vi "Get_Set_Buttons.vi"(8 "Status/Errors in":refnum<vi>, 9 "Set?":T1, 10 "Main parameters":T3={"Mode"={"Mode"=enum."Dialog", "Expert?"=FALSE, "Dialog?"=FALSE}, "Stop loop"={"Settings changed?"=FALSE, "Stop?"=refnum}, "Send message"={"Send mode"=enum."Get parameters", "Set parameter list"=0, "Get parameter list"=0, "Reset device"=0, "Length set settings message"=0, "Reset buttons?"=FALSE, "Reset Master?"=enum."General"}, "Write settings"={"Options"=enum."File 1"}, "Settings state"={"MAS locked?"=refnum, "SLV locked?"=refnum}, "Button refs"={"Stop program"=refnum, "Save settings"=refnum, "DAQ mode"=refnum, "Reset settings"=refnum, "Apply settings"=refnum, "Reset MAS"=refnum, "Reset SLV"=refnum, "Local DBase?"=refnum, "Last value DBase"=FALSE, "Database"=refnum, "Calibration"=refnum, "Save settings 2"=refnum}, "Update screen"={"Detector number"=0, "Hardware"=enum."None"}, "Files"={"Path config file"=path "", "Path def. ini file"=path "", "Path ini file 1"=path "", "Path ini file 2"=path "", "Path RBF file"=path ""}, "DB connection"={"connection reference"=refnum, "Connected?"=refnum, "ODBC Name"=""}, "Status_id"=refnum, "Time difference"=refnum, "Satellites"=refnum, "Alignment parameters"=refnum, "Page Statistics 2"=refnum, "Database"=refnum, "Page Statistics"=refnum} {"Update screen"."Detector number" format="%#.0f"; "Send message"."Reset device" format="%x"; "Send message"."Get parameter list" format="%x"; "Send message"."Set parameter list" format="%x"}) -> (0 "Status/Errors out":refnum<vi>, 1 "Button values":T2 caption="Buttons", 2 "Enabled State Expert":u8, 3 "Enabled State Normal":u8, 4 "Calibration value":bool, 5 "DAQ mode value":bool)   [LabVIEW 2013]
uses:
  Controls/Main_Parameters.ctl
  Controls/Mode.ctl
  Controls/Stop_Loop.ctl
  Controls/Send_Message.ctl
  Controls/Send_Message_Mode.ctl
  Controls/Master.ctl
  Controls/Write_Settings.ctl
  Controls/Write_Settings_Options.ctl
  Controls/Settings_State.ctl
  Controls/Button_Refs.ctl
  Controls/Update_Screen.ctl
  Controls/Files.ctl
  Controls/DB_Connection.ctl
  database/Connection.llb/Conn ObjectReference.ctl
  Controls/Button_Values.ctl
  Controls/Get_Set_Buttons_mode.ctl
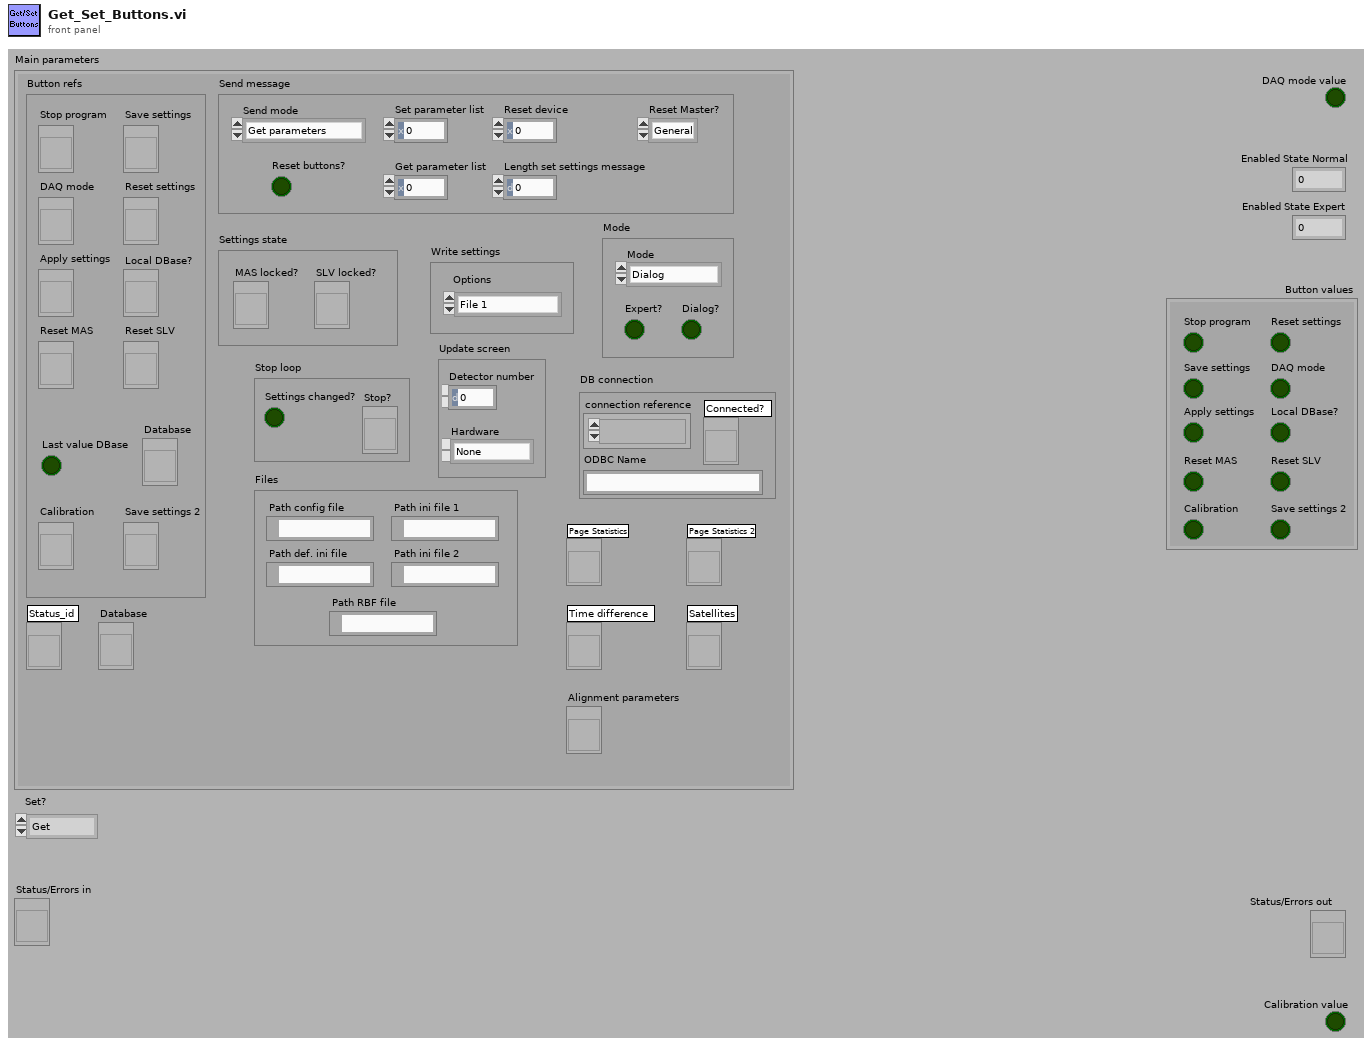
[diagram p1: front panel]
types:
  T1 = typedef "Get_Set_Buttons_mode.ctl" = enum16{"Get", "Get DAQ", "Set", "Set settings"}
  T2 = typedef "Button_Values.ctl" = cluster{"Stop program":bool, "Save settings":bool, "Apply settings":bool, "Reset settings":bool, "DAQ mode":bool, "Reset MAS":bool, "Reset SLV":bool, "Local DBase?":bool, "Calibration":bool, "Save settings 2":bool}
  T3 = typedef "Main_Parameters.ctl" = cluster{"Mode":T4, "Stop loop":T5, "Send message":T6, "Write settings":T9, "Settings state":T11, "Button refs":T12, "Update screen":T13, "Files":T14, "DB connection":T15, "Status_id":refnum<vi>, "Time difference":refnum<vi>, "Satellites":refnum<vi>, "Alignment parameters":refnum<vi>, "Page Statistics 2":refnum<vi>, "Database":refnum<vi>, "Page Statistics":refnum<vi>}
  T4 = typedef "Mode.ctl" = cluster{"Mode":enum8{"Stop", "Dialog", "Hisparc II", "Hisparc II DAQ", "Alignment"}, "Expert?":bool, "Dialog?":bool}
  T5 = typedef "Stop_Loop.ctl" = cluster{"Settings changed?":bool, "Stop?":refnum<vi>}
  T6 = typedef "Send_Message.ctl" = cluster{"Send mode":T7, "Set parameter list":u8, "Get parameter list":u8, "Reset device":u8, "Length set settings message":i32, "Reset buttons?":bool, "Reset Master?":T8}
  T7 = typedef "Send_Message_Mode.ctl" = enum16{"Get parameters", "Set parameters", "From front panel", "From parameters", "Reset device", "Alignment"}
  T8 = typedef "Master.ctl" = enum16{"Master", "Slave", "General"}
  T9 = typedef "Write_Settings.ctl" = cluster{"Options":T10}
  T10 = typedef "Write_Settings_Options.ctl" = enum16{"File 1", "File 2", "Alignment", "Reset"}
  T11 = typedef "Settings_State.ctl" = cluster{"MAS locked?":refnum<vi>, "SLV locked?":refnum<vi>}
  T12 = typedef "Button_Refs.ctl" = cluster{"Stop program":refnum<vi>, "Save settings":refnum<vi>, "DAQ mode":refnum<vi>, "Reset settings":refnum<vi>, "Apply settings":refnum<vi>, "Reset MAS":refnum<vi>, "Reset SLV":refnum<vi>, "Local DBase?":refnum<vi>, "Last value DBase":bool, "Database":refnum<vi>, "Calibration":refnum<vi>, "Save settings 2":refnum<vi>}
  T13 = typedef "Update_Screen.ctl" = cluster{"Detector number":u16, "Hardware":enum8{"None", "HiSPARC I", "HiSPARC II", "HiSPARC III", "Unknown"}}
  T14 = typedef "Files.ctl" = cluster{"Path config file":path, "Path def. ini file":path, "Path ini file 1":path, "Path ini file 2":path, "Path RBF file":path}
  T15 = typedef "DB_Connection.ctl" = cluster{"connection reference":T16, "Connected?":refnum<vi>, "ODBC Name":string}
  T16 = typedef "Conn ObjectReference.ctl" = refnum<k1>
  T17 = enum8{"Stop", "Dialog", "Hisparc II", "Hisparc II DAQ", "Alignment"}
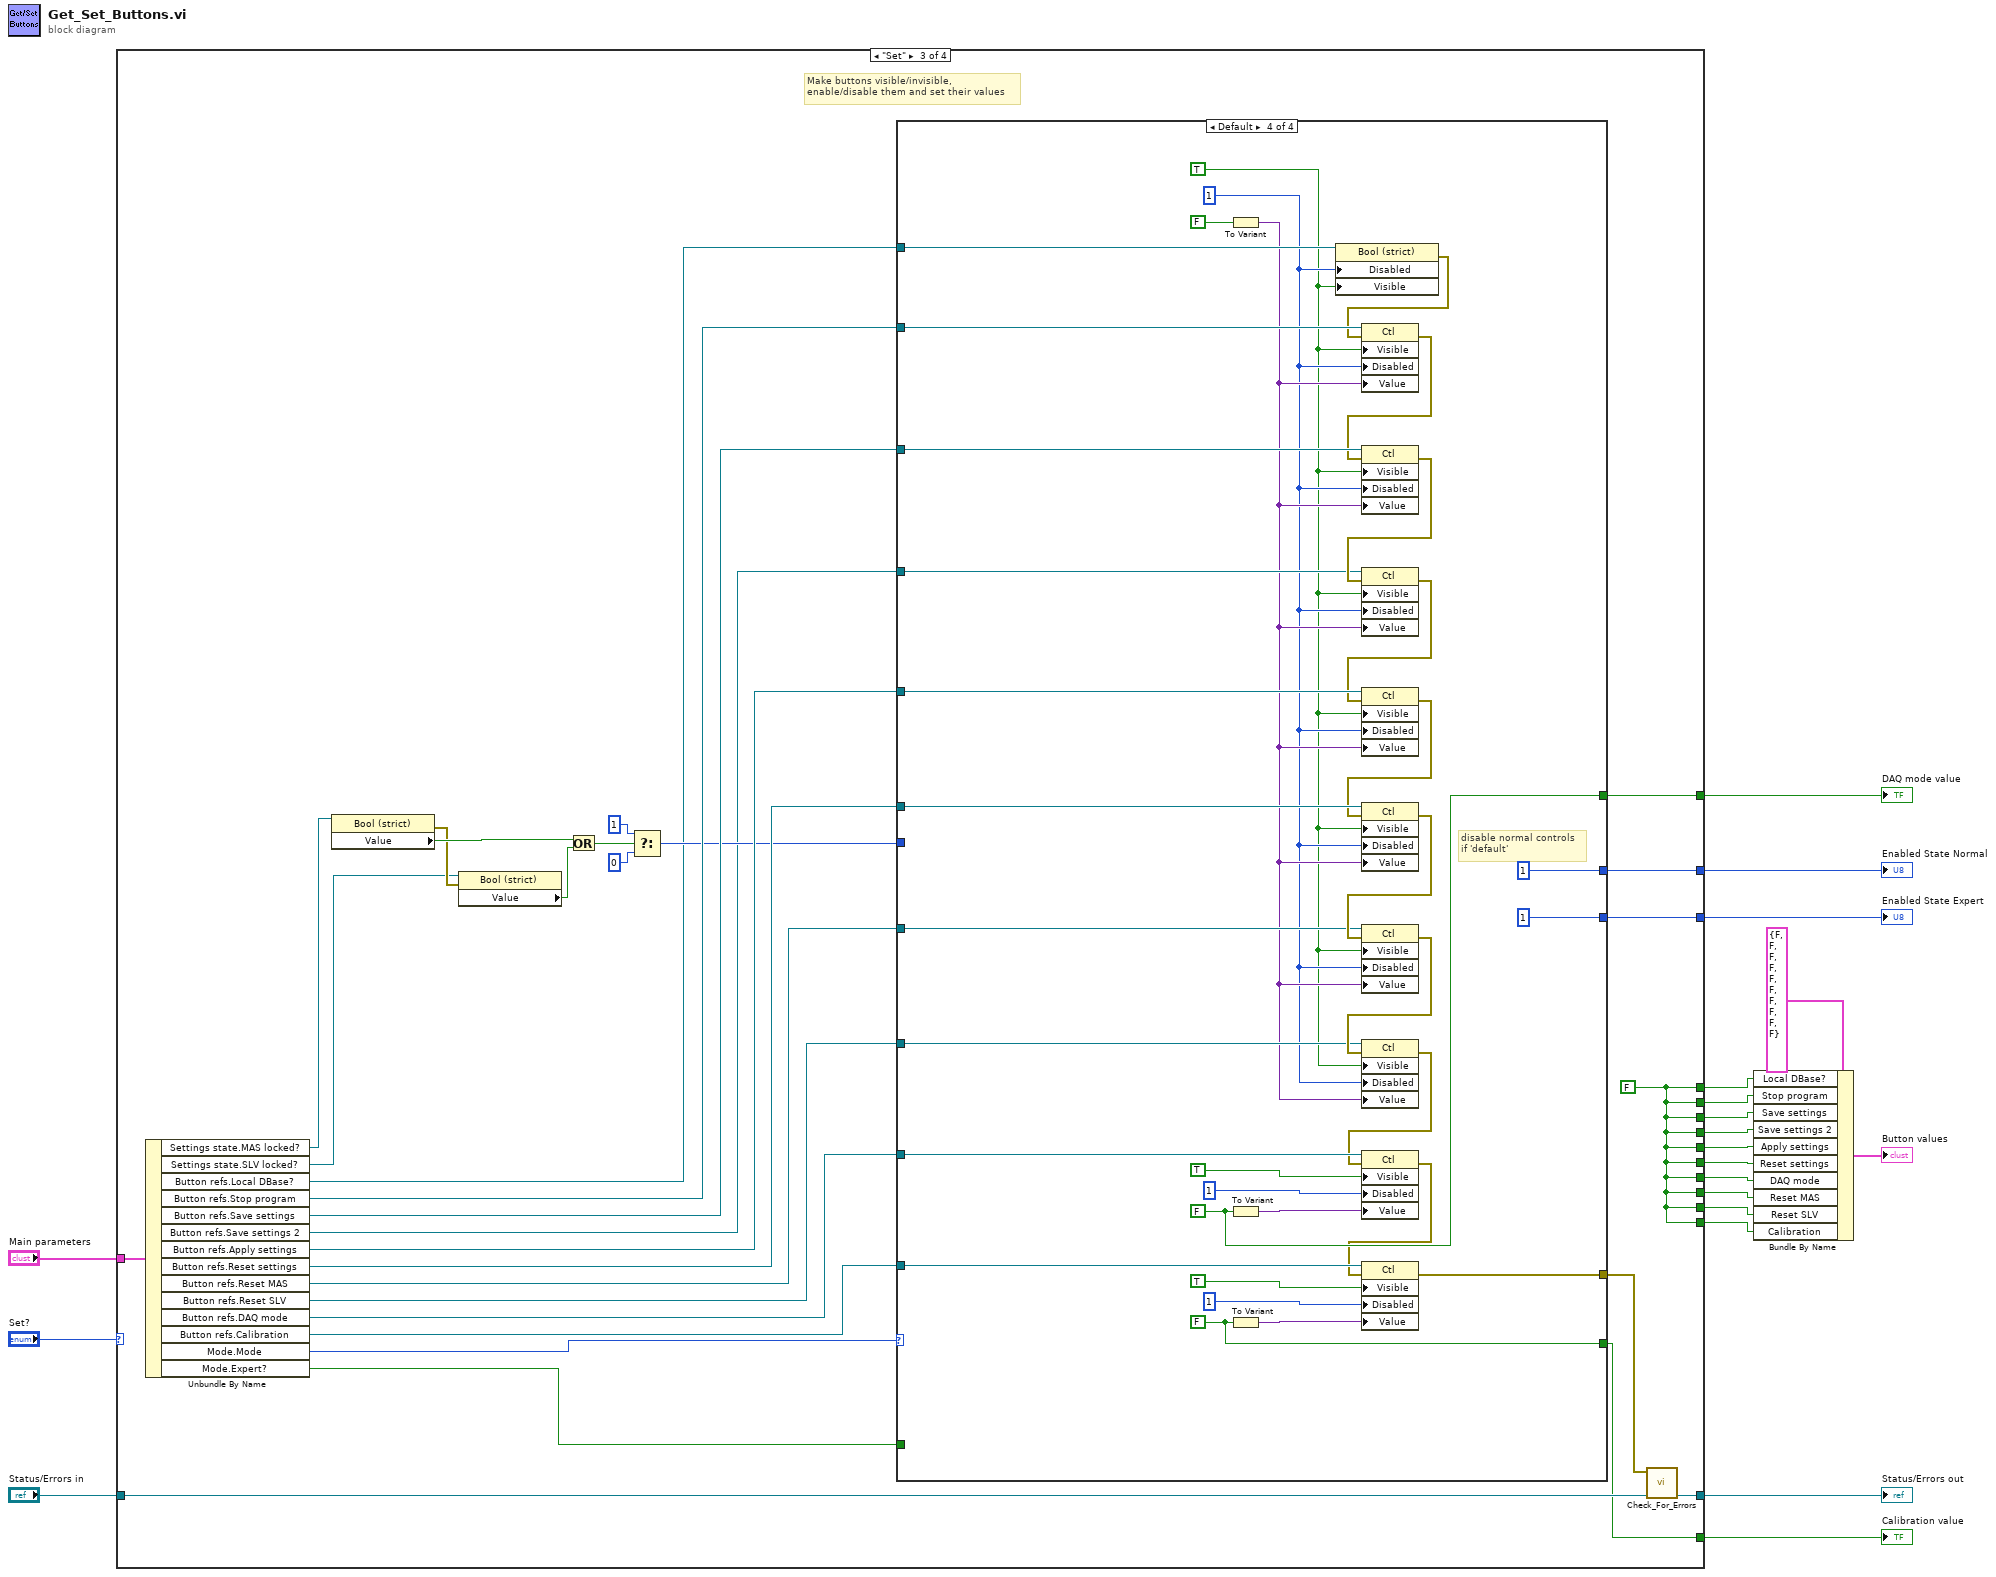
[diagram p0: block diagram]
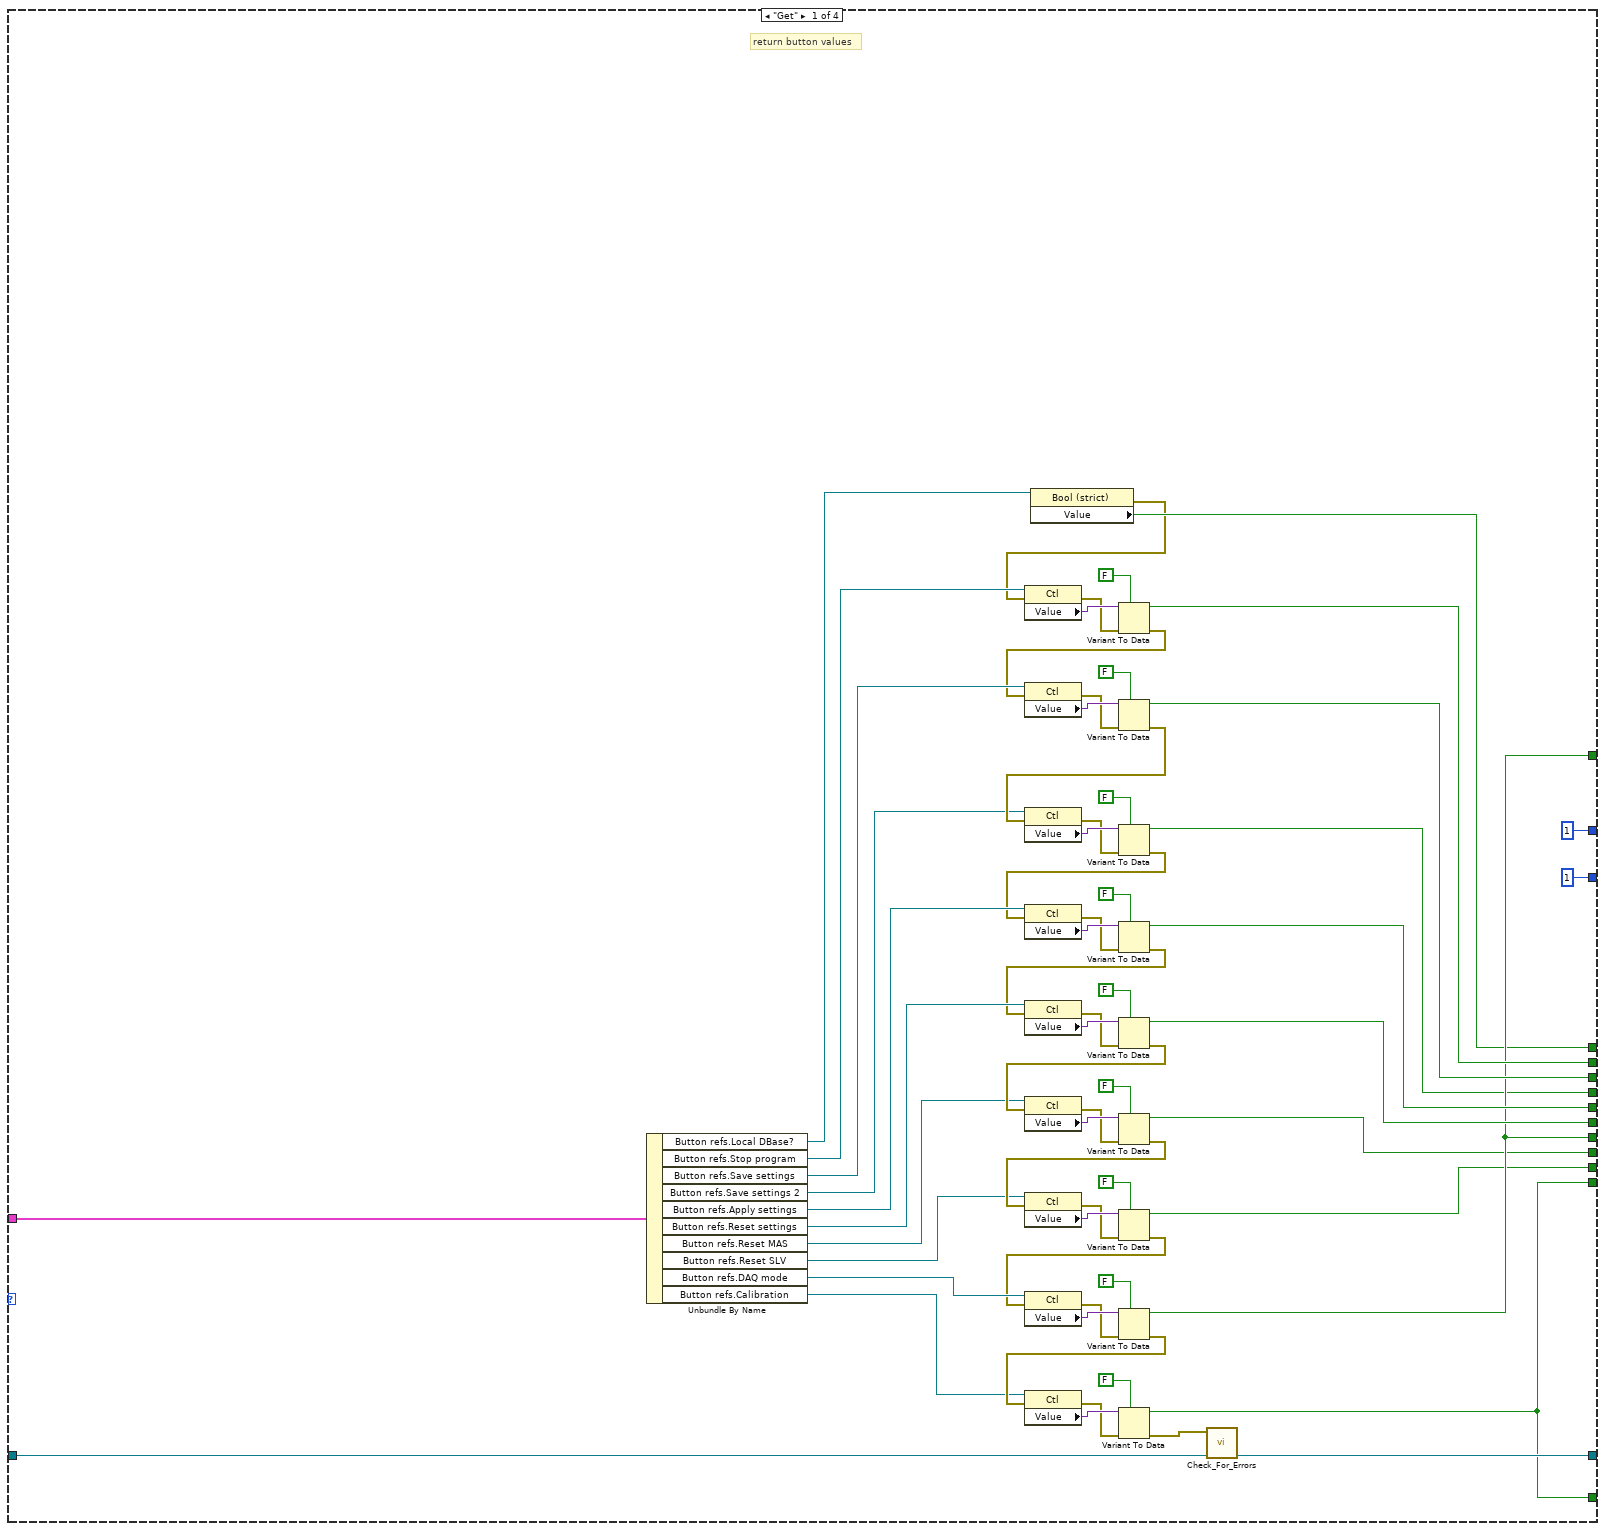
[diagram p2: hidden frame]
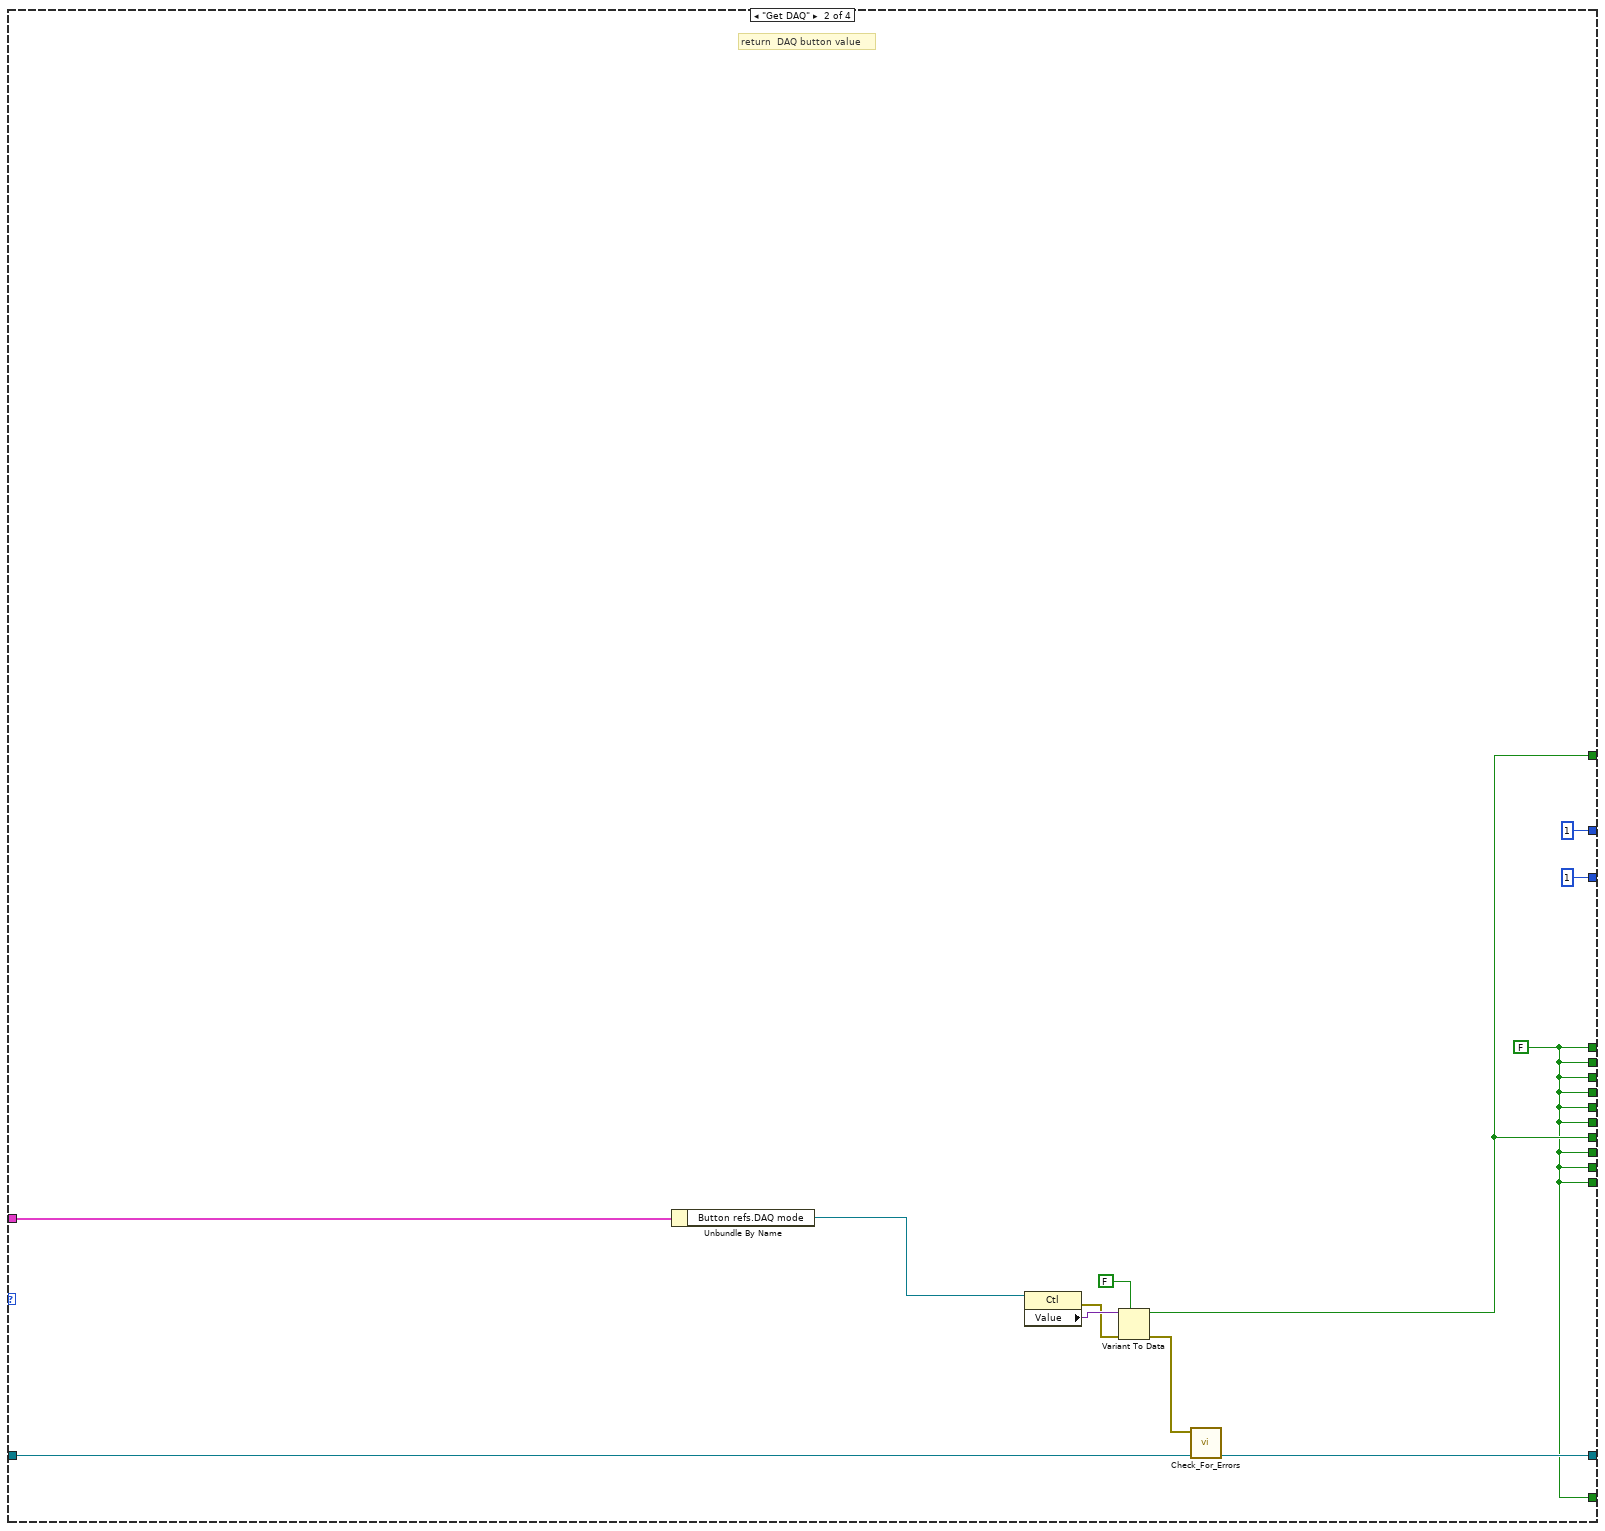
[diagram p3: hidden frame]
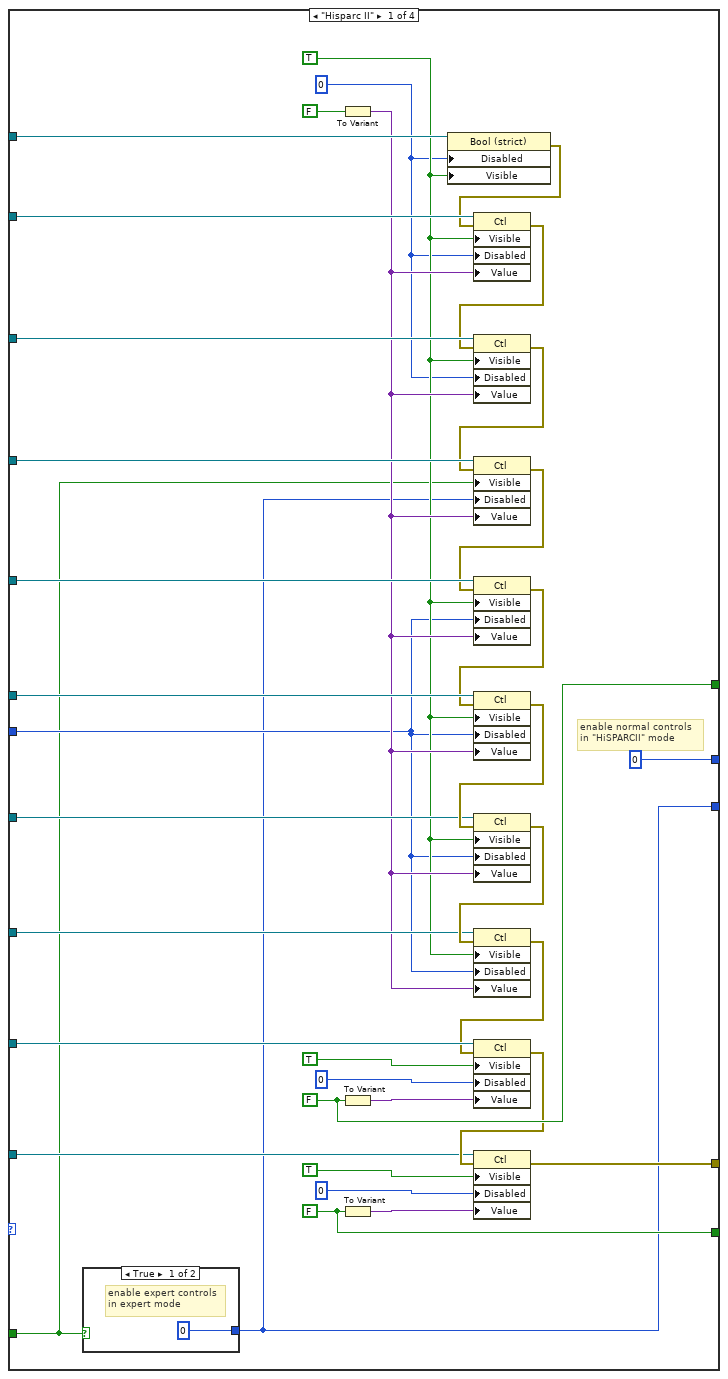
[diagram p4: hidden frame]
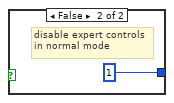
[diagram p5: hidden frame]
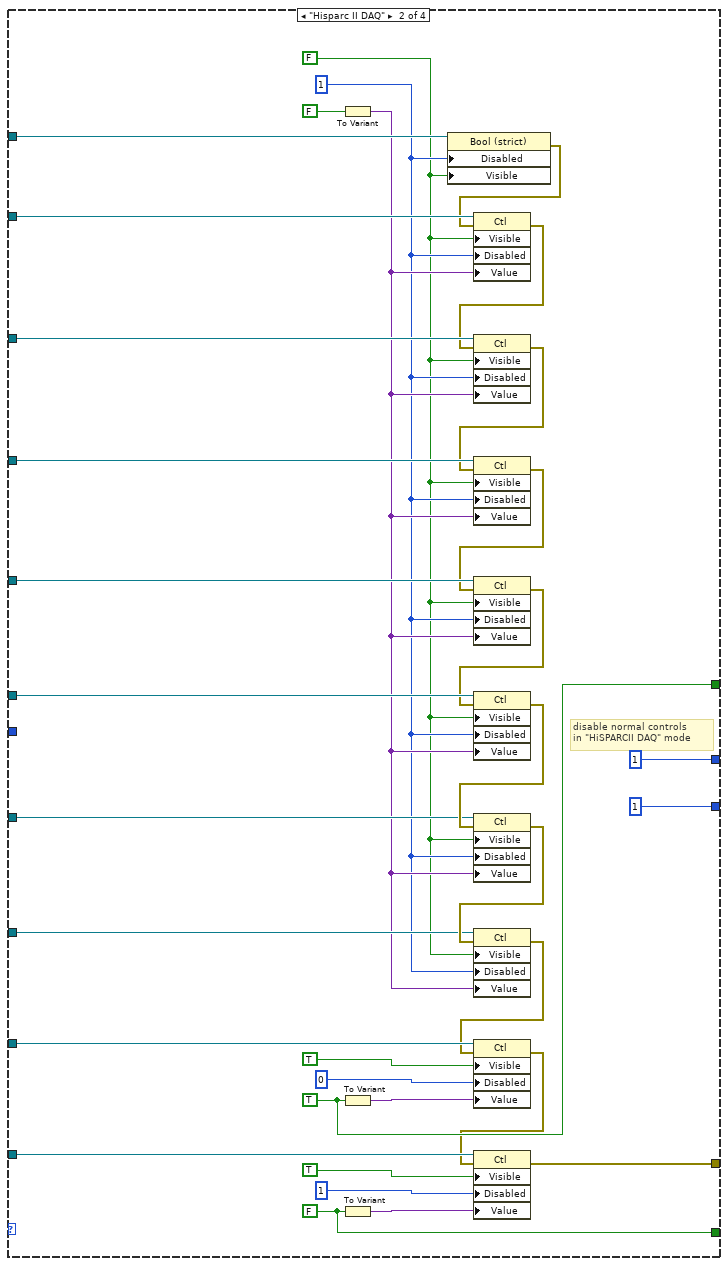
[diagram p6: hidden frame]
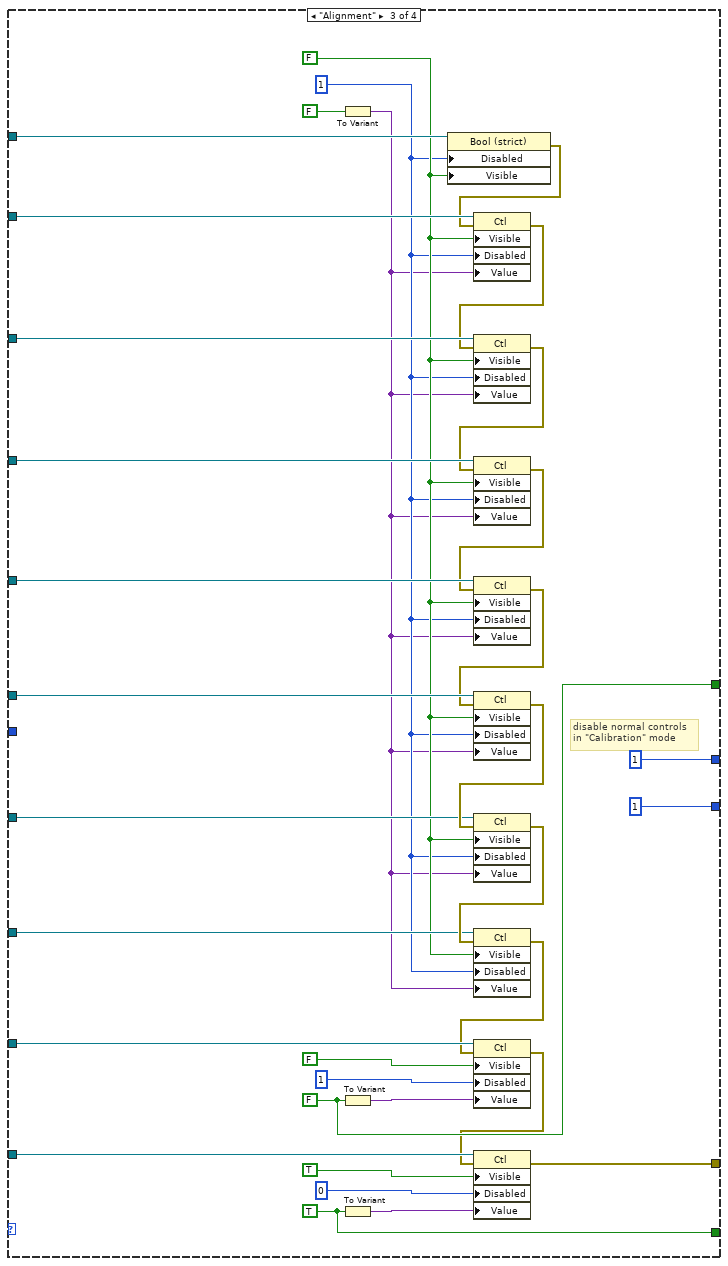
[diagram p7: hidden frame]
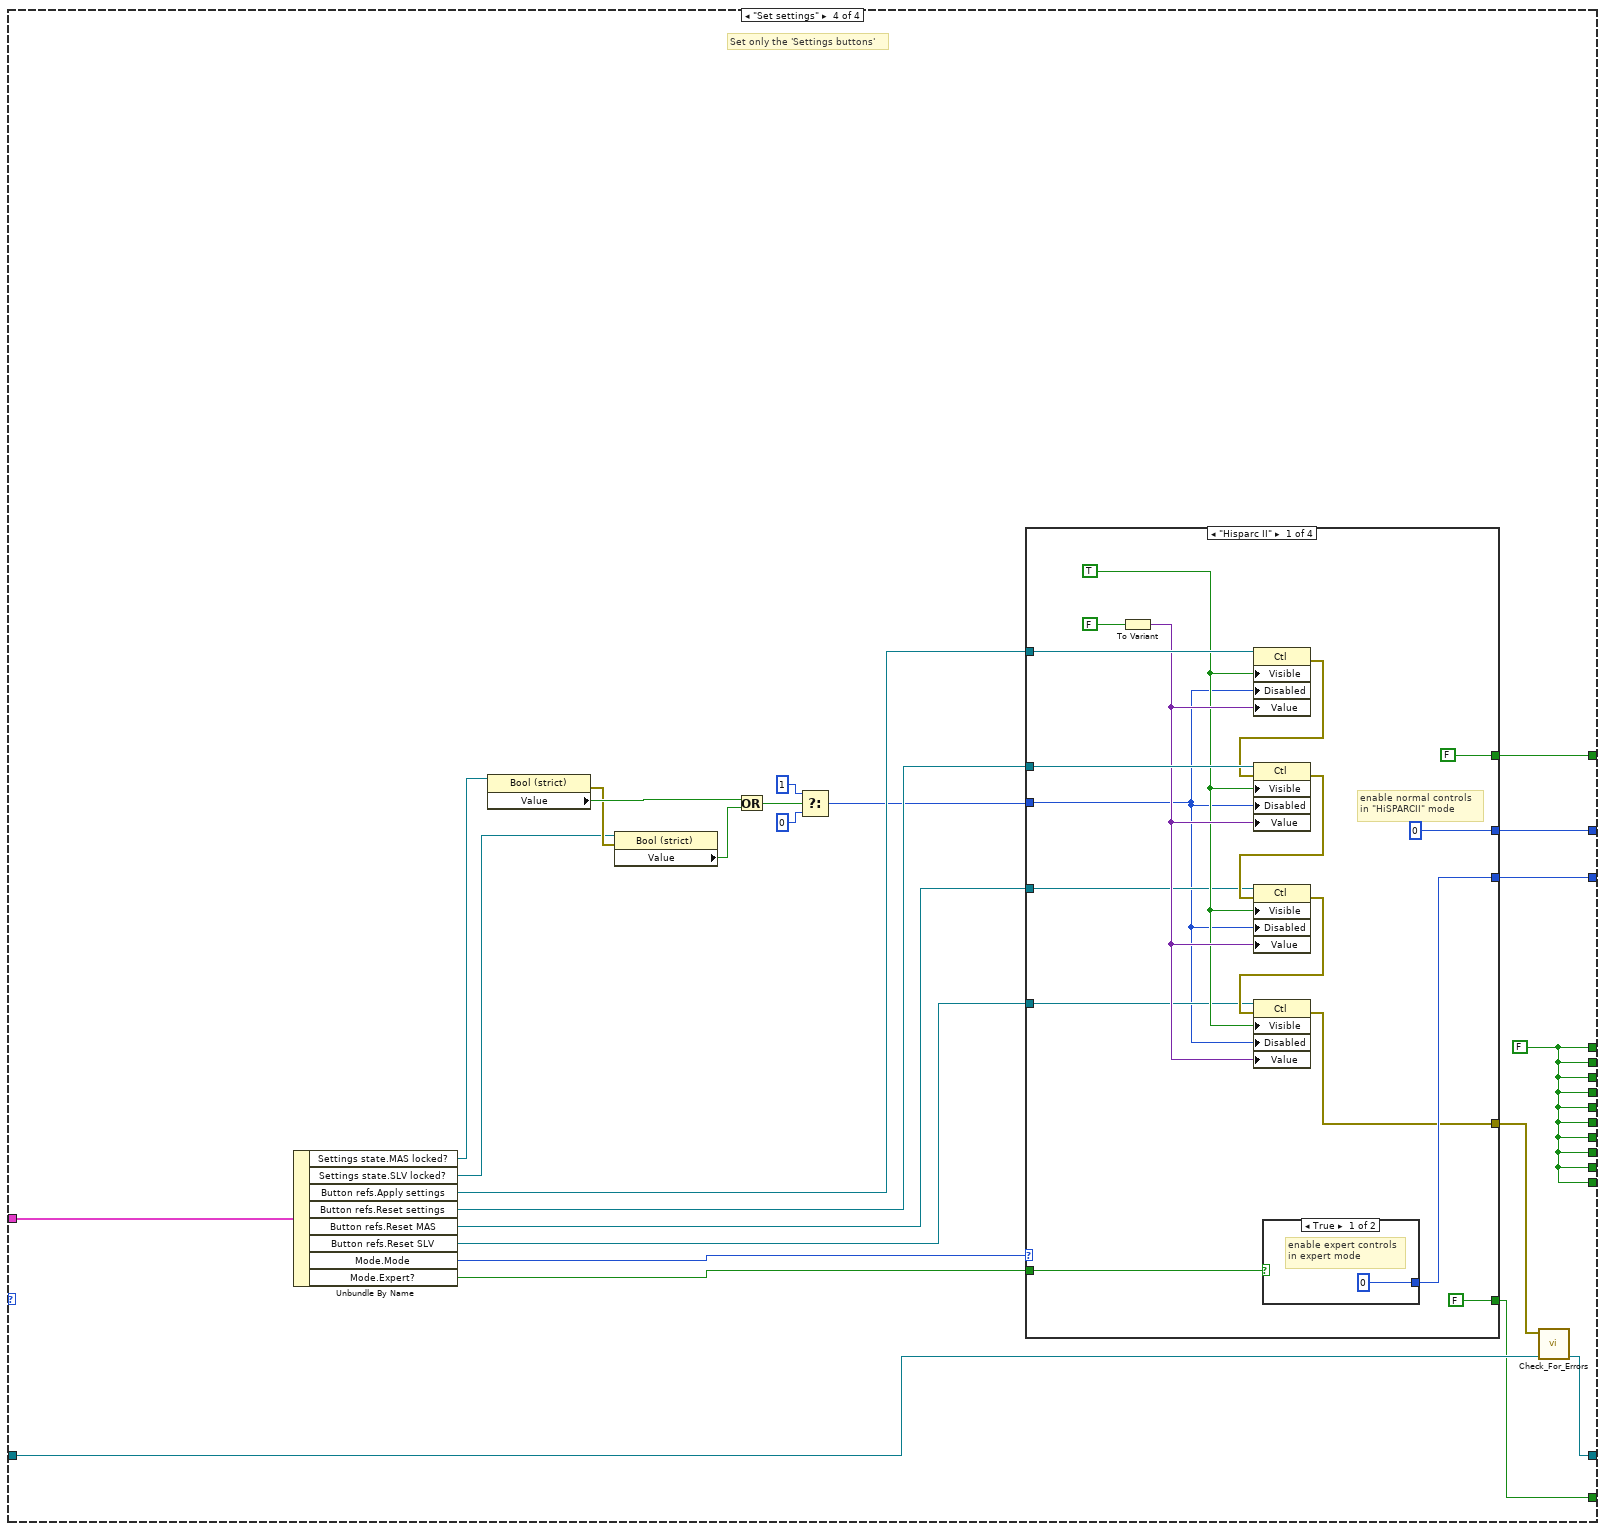
[diagram p8: hidden frame]
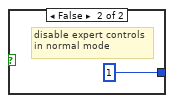
[diagram p9: hidden frame]
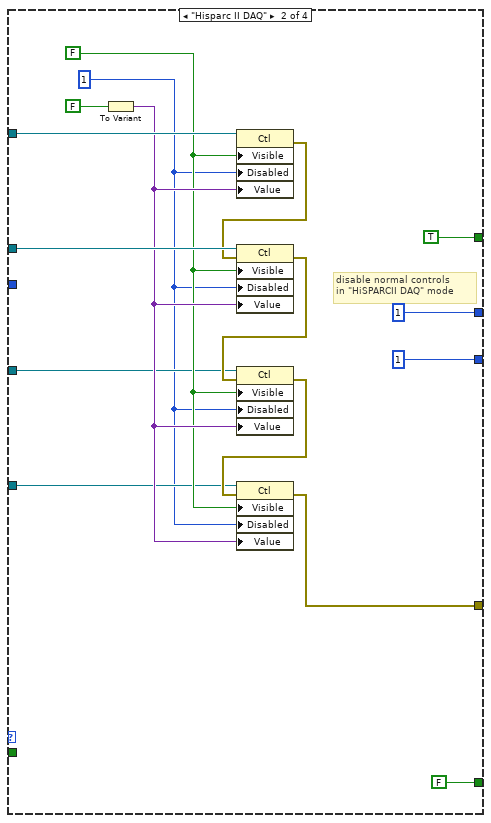
[diagram p10: hidden frame]
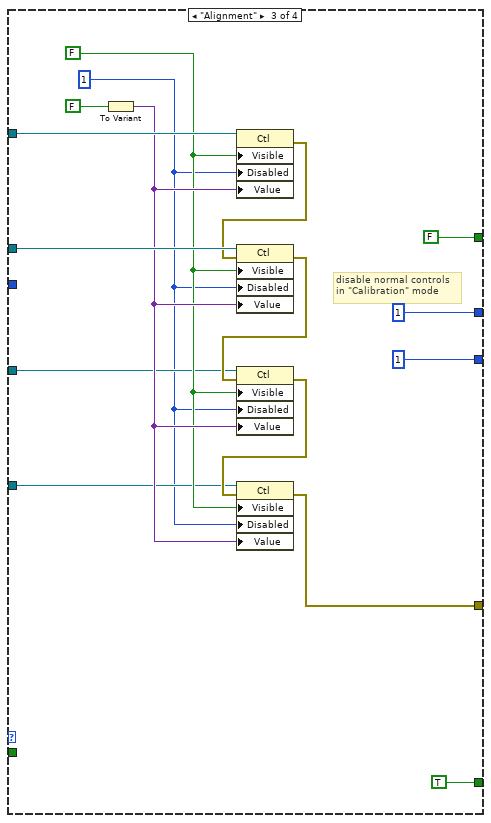
[diagram p11: hidden frame]
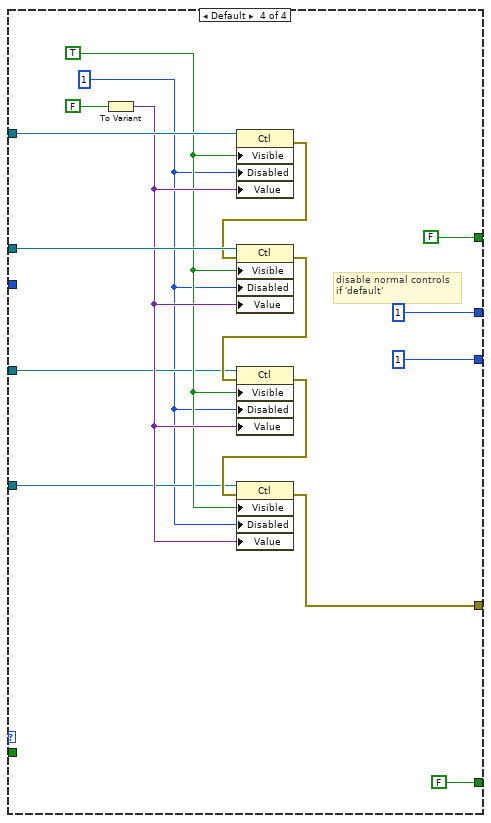
[diagram p12: hidden frame]
diagram:
  n1 = case shown="\"Set\"" "Set?" {
    tunnel: [u8 1 ("Disabled") u8 1 ("Disabled") w124 w288] -> w20
    tunnel: [u8 1 ("Disabled") u8 1 ("Disabled") w123 w287] -> w19
    tunnel: [w69 w91 w120 w284] -> w18
    tunnel: "Status/Errors in" -> [w68 w90 w119 w283]
    tunnel: "Main parameters" -> [w82 w94 w117 w281]
    tunnel: [w78 w83 w95 w265] -> w12
    tunnel: [w56 w83 w95 w265] -> w11
    tunnel: [w55 w83 w95 w265] -> w10
    tunnel: [w54 w83 w95 w265] -> w9
    tunnel: [w51 w84 w95 w265] -> w8
    tunnel: [w51 w84 w100 w267] -> w7
    tunnel: [w39 w83 w95 w265] -> w6
    tunnel: [w38 w83 w95 w265] -> w5
    tunnel: [w36 w83 w95 w265] -> w4
    tunnel: [w29 w83 w95 w265] -> w3
    tunnel: [w29 w83 w97 w266] -> w2
    tunnel: [w21 w83 w95 w265] -> w1
    frame "Get" {
      # "return button values"
      n2 = Unbundle By Name(w82) -> ("Button refs.Local DBase?"=w37:refnum<vi>, "Button refs.Stop program"=w81:refnum<vi>, "Button refs.Save settings"=w67:refnum<vi>, "Button refs.Save settings 2"=w22:refnum<vi>, "Button refs.Apply settings"=w66:refnum<vi>, "Button refs.Reset settings"=w65:refnum<vi>, "Button refs.Reset MAS"=w41:refnum<vi>, "Button refs.Reset SLV"=w40:refnum<vi>, "Button refs.DAQ mode"=w64:refnum<vi>, "Button refs.Calibration"=w28:refnum<vi>)
      n3 = property class="Bool (strict)"(reference=w37) -> (error out=w35:errorcluster, "Value"=w36:bool)  [unwired: 1 in, 1 out]
      n4 = property class="Ctl"(reference=w81, error in=w35) -> (error out=w59:errorcluster, "Value"=w80:variant)  [unwired: 1 out]
      n5 = Variant To Data(error in=w59, type=FALSE, Variant=w80) -> (data=w78:bool, error out=w58:errorcluster)
      n6 = property class="Ctl"(reference=w67, error in=w58) -> (error out=w60:errorcluster, "Value"=w77:variant)  [unwired: 1 out]
      n7 = Variant To Data(error in=w60, type=FALSE, Variant=w77) -> (data=w56:bool, error out=w24:errorcluster)
      n8 = property class="Ctl"(reference=w22, error in=w24) -> (error out=w25:errorcluster, "Value"=w27:variant)  [unwired: 1 out]
      n9 = Variant To Data(error in=w25, type=FALSE, Variant=w27) -> (data=w21:bool, error out=w23:errorcluster)
      n10 = property class="Ctl"(reference=w66, error in=w23) -> (error out=w61:errorcluster, "Value"=w75:variant)  [unwired: 1 out]
      n11 = Variant To Data(error in=w61, type=FALSE, Variant=w75) -> (data=w55:bool, error out=w57:errorcluster)
      n12 = property class="Ctl"(reference=w65, error in=w57) -> (error out=w62:errorcluster, "Value"=w73:variant)  [unwired: 1 out]
      n13 = Variant To Data(error in=w62, type=FALSE, Variant=w73) -> (data=w54:bool, error out=w44:errorcluster)
      n14 = property class="Ctl"(reference=w41, error in=w44) -> (error out=w45:errorcluster, "Value"=w50:variant)  [unwired: 1 out]
      n15 = Variant To Data(error in=w45, type=FALSE, Variant=w50) -> (data=w39:bool, error out=w43:errorcluster)
      n16 = property class="Ctl"(reference=w40, error in=w43) -> (error out=w46:errorcluster, "Value"=w48:variant)  [unwired: 1 out]
      n17 = Variant To Data(error in=w46, type=FALSE, Variant=w48) -> (data=w38:bool, error out=w42:errorcluster)
      n18 = property class="Ctl"(reference=w64, error in=w42) -> (error out=w63:errorcluster, "Value"=w71:variant)  [unwired: 1 out]
      n19 = Variant To Data(error in=w63, type=FALSE, Variant=w71) -> (data=w51:bool, error out=w31:errorcluster)
      n20 = property class="Ctl"(reference=w28, error in=w31) -> (error out=w32:errorcluster, "Value"=w34:variant)  [unwired: 1 out]
      n21 = Variant To Data(error in=w32, type=FALSE, Variant=w34) -> (data=w29:bool, error out=w30:errorcluster)
      n22 = call "Check_For_Errors.vi"("Status/Errors in"=w68, "error in"=w30) -> ("Status/Errors out"=w69:refnum<vi>)  [unwired: 9 out]
    }
    frame "Get DAQ" {
      w83 = FALSE
      # "return  DAQ button value"
      n23 = Unbundle By Name(w94) -> ("Button refs.DAQ mode"=w88:refnum<vi>)
      n24 = property class="Ctl"(reference=w88) -> (error out=w87:errorcluster, "Value"=w93:variant)  [unwired: 1 in, 1 out]
      n25 = Variant To Data(error in=w87, type=FALSE, Variant=w93) -> (data=w84:bool, error out=w89:errorcluster)
      n26 = call "Check_For_Errors.vi"("Status/Errors in"=w90, "error in"=w89) -> ("Status/Errors out"=w91:refnum<vi>)  [unwired: 9 out]
    }
    frame "Set" {
      w95 = FALSE
      # "Make buttons visible/invisible,\nenable/disable them and set their values"
      n27 = Unbundle By Name(w117) -> ("Settings state.MAS locked?"=w112:refnum<vi>, "Settings state.SLV locked?"=w109:refnum<vi>, "Button refs.Local DBase?"=w99:refnum<vi>, "Button refs.Stop program"=w116:refnum<vi>, "Button refs.Save settings"=w115:refnum<vi>, "Button refs.Save settings 2"=w96:refnum<vi>, "Button refs.Apply settings"=w114:refnum<vi>, "Button refs.Reset settings"=w113:refnum<vi>, "Button refs.Reset MAS"=w102:refnum<vi>, "Button refs.Reset SLV"=w101:refnum<vi>, "Button refs.DAQ mode"=w103:refnum<vi>, "Button refs.Calibration"=w98:refnum<vi>, "Mode.Mode"=w122:T17, "Mode.Expert?"=w121:bool)
      n28 = property class="Bool (strict)"(reference=w112) -> (error out=w110:errorcluster, "Value"=w111:bool)  [unwired: 1 in, 1 out]
      n29 = property class="Bool (strict)"(reference=w109, error in=w110) -> ("Value"=w108:bool)  [unwired: 2 out]
      n30 = Or(x=w111, y=w108) -> (x .or. y?=w107:bool)
      n31 = Select(t=u8 1 ("Disabled"), s=w107, f=u8 0 ("Disabled")) -> (s? t:f=w104:u8)
      n32 = case shown="Default" w122 {
        tunnel: [u8 0 ("Disabled") u8 1 ("Disabled") u8 1 ("Disabled") u8 1 ("Disabled")] -> w124
        tunnel: [w125 u8 1 ("Disabled") u8 1 ("Disabled") u8 1 ("Disabled")] -> w123
        tunnel: w116 -> [w158 w194 w228 w262]
        tunnel: w115 -> [w157 w193 w227 w261]
        tunnel: w114 -> [w156 w192 w226 w260]
        tunnel: w113 -> [w155 w191 w225 w259]
        tunnel: w103 -> [w159 w195 w229 w263]
        tunnel: [w136 w171 w205 w238] -> w118
        tunnel: w121 -> [w126 _ _ _]
        tunnel: [w148 w184 w218 w253] -> w100
        tunnel: w104 -> [w127 _ _ _]
        tunnel: w102 -> [w144 w180 w214 w249]
        tunnel: w101 -> [w143 w179 w213 w248]
        tunnel: w99 -> [w142 w177 w211 w244]
        tunnel: w98 -> [w135 w172 w206 w240]
        tunnel: [w134 w170 w204 w239] -> w97
        tunnel: w96 -> [w133 w168 w202 w235]
        frame "Hisparc II" {
          w134 = FALSE ("Visible")
          w129 = u8 0 ("Disabled")
          w130 = TRUE
          w148 = FALSE ("Visible")
          # "enable normal controls\nin \"HiSPARCII\" mode"
          n33 = case shown="True" w126 {
            tunnel: [u8 0 ("Disabled") u8 1 ("Disabled")] -> w125
            frame True {
              # "enable expert controls\nin expert mode"
            }
            frame False {
              # "disable expert controls\nin normal mode"
            }
          }
          n34 = To Variant(anything=FALSE) -> (Variant=w131:variant)
          n35 = To Variant(anything=w148) -> (Variant=w151:variant)
          n36 = To Variant(anything=w134) -> (Variant=w139:variant)
          n37 = property class="Bool (strict)"(reference=w142, "Disabled"=w129, "Visible"=w130) -> (error out=w141:errorcluster)  [unwired: 1 in, 1 out]
          n38 = property class="Ctl"(reference=w158, error in=w141, "Visible"=w130, "Disabled"=w129, "Value"=w131) -> (error out=w153:errorcluster)  [unwired: 1 out]
          n39 = property class="Ctl"(reference=w157, error in=w153, "Visible"=w130, "Disabled"=w129, "Value"=w131) -> (error out=w132:errorcluster)  [unwired: 1 out]
          n40 = property class="Ctl"(reference=w133, error in=w132, "Visible"=w126, "Disabled"=w125, "Value"=w131) -> (error out=w128:errorcluster)  [unwired: 1 out]
          n41 = property class="Ctl"(reference=w156, error in=w128, "Visible"=w130, "Disabled"=w127, "Value"=w131) -> (error out=w152:errorcluster)  [unwired: 1 out]
          n42 = property class="Ctl"(reference=w155, error in=w152, "Visible"=w130, "Disabled"=w127, "Value"=w131) -> (error out=w146:errorcluster)  [unwired: 1 out]
          n43 = property class="Ctl"(reference=w144, error in=w146, "Visible"=w130, "Disabled"=w127, "Value"=w131) -> (error out=w147:errorcluster)  [unwired: 1 out]
          n44 = property class="Ctl"(reference=w143, error in=w147, "Visible"=w130, "Disabled"=w127, "Value"=w131) -> (error out=w145:errorcluster)  [unwired: 1 out]
          n45 = property class="Ctl"(reference=w159, error in=w145, "Visible"=TRUE, "Disabled"=u8 0, "Value"=w151) -> (error out=w137:errorcluster)  [unwired: 1 out]
          n46 = property class="Ctl"(reference=w135, error in=w137, "Visible"=TRUE, "Disabled"=u8 0, "Value"=w139) -> (error out=w136:errorcluster)  [unwired: 1 out]
        }
        frame "Hisparc II DAQ" {
          w170 = FALSE ("Visible")
          w165 = u8 1 ("Disabled")
          w164 = FALSE
          w184 = TRUE ("Visible")
          # "disable normal controls\nin \"HiSPARCII DAQ\" mode"
          n47 = To Variant(anything=FALSE) -> (Variant=w166:variant)
          n48 = To Variant(anything=w184) -> (Variant=w187:variant)
          n49 = To Variant(anything=w170) -> (Variant=w174:variant)
          n50 = property class="Bool (strict)"(reference=w177, "Disabled"=w165, "Visible"=w164) -> (error out=w176:errorcluster)  [unwired: 1 in, 1 out]
          n51 = property class="Ctl"(reference=w194, error in=w176, "Visible"=w164, "Disabled"=w165, "Value"=w166) -> (error out=w189:errorcluster)  [unwired: 1 out]
          n52 = property class="Ctl"(reference=w193, error in=w189, "Visible"=w164, "Disabled"=w165, "Value"=w166) -> (error out=w167:errorcluster)  [unwired: 1 out]
          n53 = property class="Ctl"(reference=w168, error in=w167, "Visible"=w164, "Disabled"=w165, "Value"=w166) -> (error out=w163:errorcluster)  [unwired: 1 out]
          n54 = property class="Ctl"(reference=w192, error in=w163, "Visible"=w164, "Disabled"=w165, "Value"=w166) -> (error out=w188:errorcluster)  [unwired: 1 out]
          n55 = property class="Ctl"(reference=w191, error in=w188, "Visible"=w164, "Disabled"=w165, "Value"=w166) -> (error out=w182:errorcluster)  [unwired: 1 out]
          n56 = property class="Ctl"(reference=w180, error in=w182, "Visible"=w164, "Disabled"=w165, "Value"=w166) -> (error out=w183:errorcluster)  [unwired: 1 out]
          n57 = property class="Ctl"(reference=w179, error in=w183, "Visible"=w164, "Disabled"=w165, "Value"=w166) -> (error out=w181:errorcluster)  [unwired: 1 out]
          n58 = property class="Ctl"(reference=w195, error in=w181, "Visible"=TRUE, "Disabled"=u8 0, "Value"=w187) -> (error out=w169:errorcluster)  [unwired: 1 out]
          n59 = property class="Ctl"(reference=w172, error in=w169, "Visible"=TRUE, "Disabled"=u8 1, "Value"=w174) -> (error out=w171:errorcluster)  [unwired: 1 out]
        }
        frame "Alignment" {
          w204 = TRUE ("Visible")
          w199 = u8 1 ("Disabled")
          w200 = FALSE
          w218 = FALSE ("Visible")
          # "disable normal controls\nin \"Calibration\" mode"
          n60 = To Variant(anything=FALSE) -> (Variant=w198:variant)
          n61 = To Variant(anything=w218) -> (Variant=w221:variant)
          n62 = To Variant(anything=w204) -> (Variant=w208:variant)
          n63 = property class="Bool (strict)"(reference=w211, "Disabled"=w199, "Visible"=w200) -> (error out=w210:errorcluster)  [unwired: 1 in, 1 out]
          n64 = property class="Ctl"(reference=w228, error in=w210, "Visible"=w200, "Disabled"=w199, "Value"=w198) -> (error out=w223:errorcluster)  [unwired: 1 out]
          n65 = property class="Ctl"(reference=w227, error in=w223, "Visible"=w200, "Disabled"=w199, "Value"=w198) -> (error out=w201:errorcluster)  [unwired: 1 out]
          n66 = property class="Ctl"(reference=w202, error in=w201, "Visible"=w200, "Disabled"=w199, "Value"=w198) -> (error out=w197:errorcluster)  [unwired: 1 out]
          n67 = property class="Ctl"(reference=w226, error in=w197, "Visible"=w200, "Disabled"=w199, "Value"=w198) -> (error out=w222:errorcluster)  [unwired: 1 out]
          n68 = property class="Ctl"(reference=w225, error in=w222, "Visible"=w200, "Disabled"=w199, "Value"=w198) -> (error out=w216:errorcluster)  [unwired: 1 out]
          n69 = property class="Ctl"(reference=w214, error in=w216, "Visible"=w200, "Disabled"=w199, "Value"=w198) -> (error out=w217:errorcluster)  [unwired: 1 out]
          n70 = property class="Ctl"(reference=w213, error in=w217, "Visible"=w200, "Disabled"=w199, "Value"=w198) -> (error out=w215:errorcluster)  [unwired: 1 out]
          n71 = property class="Ctl"(reference=w229, error in=w215, "Visible"=FALSE, "Disabled"=u8 1, "Value"=w221) -> (error out=w203:errorcluster)  [unwired: 1 out]
          n72 = property class="Ctl"(reference=w206, error in=w203, "Visible"=TRUE, "Disabled"=u8 0, "Value"=w208) -> (error out=w205:errorcluster)  [unwired: 1 out]
        }
        frame Default {
          w239 = FALSE ("Visible")
          w232 = u8 1 ("Disabled")
          w231 = TRUE
          w253 = FALSE ("Visible")
          # "disable normal controls\nif 'default'"
          n73 = To Variant(anything=FALSE) -> (Variant=w233:variant)
          n74 = To Variant(anything=w253) -> (Variant=w256:variant)
          n75 = To Variant(anything=w239) -> (Variant=w242:variant)
          n76 = property class="Bool (strict)"(reference=w244, "Disabled"=w232, "Visible"=w231) -> (error out=w246:errorcluster)  [unwired: 1 in, 1 out]
          n77 = property class="Ctl"(reference=w262, error in=w246, "Visible"=w231, "Disabled"=w232, "Value"=w233) -> (error out=w245:errorcluster)  [unwired: 1 out]
          n78 = property class="Ctl"(reference=w261, error in=w245, "Visible"=w231, "Disabled"=w232, "Value"=w233) -> (error out=w236:errorcluster)  [unwired: 1 out]
          n79 = property class="Ctl"(reference=w235, error in=w236, "Visible"=w231, "Disabled"=w232, "Value"=w233) -> (error out=w234:errorcluster)  [unwired: 1 out]
          n80 = property class="Ctl"(reference=w260, error in=w234, "Visible"=w231, "Disabled"=w232, "Value"=w233) -> (error out=w257:errorcluster)  [unwired: 1 out]
          n81 = property class="Ctl"(reference=w259, error in=w257, "Visible"=w231, "Disabled"=w232, "Value"=w233) -> (error out=w251:errorcluster)  [unwired: 1 out]
          n82 = property class="Ctl"(reference=w249, error in=w251, "Visible"=w231, "Disabled"=w232, "Value"=w233) -> (error out=w252:errorcluster)  [unwired: 1 out]
          n83 = property class="Ctl"(reference=w248, error in=w252, "Visible"=w231, "Disabled"=w232, "Value"=w233) -> (error out=w250:errorcluster)  [unwired: 1 out]
          n84 = property class="Ctl"(reference=w263, error in=w250, "Visible"=TRUE, "Disabled"=u8 1, "Value"=w256) -> (error out=w237:errorcluster)  [unwired: 1 out]
          n85 = property class="Ctl"(reference=w240, error in=w237, "Visible"=TRUE, "Disabled"=u8 1, "Value"=w242) -> (error out=w238:errorcluster)  [unwired: 1 out]
        }
      }
      n86 = call "Check_For_Errors.vi"("Status/Errors in"=w119, "error in"=w118) -> ("Status/Errors out"=w120:refnum<vi>)  [unwired: 9 out]
    }
    frame "Set settings" {
      w265 = FALSE
      # "Set only the 'Settings buttons'"
      n87 = Unbundle By Name(w281) -> ("Settings state.MAS locked?"=w278:refnum<vi>, "Settings state.SLV locked?"=w275:refnum<vi>, "Button refs.Apply settings"=w280:refnum<vi>, "Button refs.Reset settings"=w279:refnum<vi>, "Button refs.Reset MAS"=w269:refnum<vi>, "Button refs.Reset SLV"=w268:refnum<vi>, "Mode.Mode"=w286:T17, "Mode.Expert?"=w285:bool)
      n88 = property class="Bool (strict)"(reference=w278) -> (error out=w276:errorcluster, "Value"=w277:bool)  [unwired: 1 in, 1 out]
      n89 = property class="Bool (strict)"(reference=w275, error in=w276) -> ("Value"=w274:bool)  [unwired: 2 out]
      n90 = Or(x=w277, y=w274) -> (x .or. y?=w273:bool)
      n91 = Select(t=u8 1 ("Disabled"), s=w273, f=u8 0 ("Disabled")) -> (s? t:f=w270:u8)
      n92 = case shown="\"Hisparc II\"" w286 {
        tunnel: [u8 0 ("Disabled") u8 1 ("Disabled") u8 1 ("Disabled") u8 1 ("Disabled")] -> w288
        tunnel: [w304 u8 1 ("Disabled") u8 1 ("Disabled") u8 1 ("Disabled")] -> w287
        tunnel: w280 -> [w302 w322 w338 w354]
        tunnel: w279 -> [w301 w321 w337 w353]
        tunnel: [w291 w310 w326 w342] -> w282
        tunnel: w285 -> [w303 _ _ _]
        tunnel: [FALSE ("Visible") TRUE ("Visible") FALSE ("Visible") FALSE ("Visible")] -> w267
        tunnel: w270 -> [w292 _ _ _]
        tunnel: w269 -> [w294 w314 w330 w346]
        tunnel: w268 -> [w293 w313 w329 w345]
        tunnel: [FALSE FALSE TRUE FALSE] -> w266
        frame "Hisparc II" {
          w295 = TRUE
          # "enable normal controls\nin \"HiSPARCII\" mode"
          n93 = To Variant(anything=FALSE) -> (Variant=w296:variant)
          n94 = property class="Ctl"(reference=w302, "Visible"=w295, "Disabled"=w292, "Value"=w296) -> (error out=w300:errorcluster)  [unwired: 1 in, 1 out]
          n95 = property class="Ctl"(reference=w301, error in=w300, "Visible"=w295, "Disabled"=w292, "Value"=w296) -> (error out=w297:errorcluster)  [unwired: 1 out]
          n96 = property class="Ctl"(reference=w294, error in=w297, "Visible"=w295, "Disabled"=w292, "Value"=w296) -> (error out=w298:errorcluster)  [unwired: 1 out]
          n97 = property class="Ctl"(reference=w293, error in=w298, "Visible"=w295, "Disabled"=w292, "Value"=w296) -> (error out=w291:errorcluster)  [unwired: 1 out]
          n98 = case shown="True" w303 {
            tunnel: [u8 0 ("Disabled") u8 1 ("Disabled")] -> w304
            frame True {
              # "enable expert controls\nin expert mode"
            }
            frame False {
              # "disable expert controls\nin normal mode"
            }
          }
        }
        frame "Hisparc II DAQ" {
          w311 = u8 1 ("Disabled")
          w315 = FALSE
          # "disable normal controls\nin \"HiSPARCII DAQ\" mode"
          n99 = To Variant(anything=FALSE) -> (Variant=w316:variant)
          n100 = property class="Ctl"(reference=w322, "Visible"=w315, "Disabled"=w311, "Value"=w316) -> (error out=w320:errorcluster)  [unwired: 1 in, 1 out]
          n101 = property class="Ctl"(reference=w321, error in=w320, "Visible"=w315, "Disabled"=w311, "Value"=w316) -> (error out=w317:errorcluster)  [unwired: 1 out]
          n102 = property class="Ctl"(reference=w314, error in=w317, "Visible"=w315, "Disabled"=w311, "Value"=w316) -> (error out=w318:errorcluster)  [unwired: 1 out]
          n103 = property class="Ctl"(reference=w313, error in=w318, "Visible"=w315, "Disabled"=w311, "Value"=w316) -> (error out=w310:errorcluster)  [unwired: 1 out]
        }
        frame "Alignment" {
          w327 = u8 1 ("Disabled")
          w331 = FALSE
          # "disable normal controls\nin \"Calibration\" mode"
          n104 = To Variant(anything=FALSE) -> (Variant=w332:variant)
          n105 = property class="Ctl"(reference=w338, "Visible"=w331, "Disabled"=w327, "Value"=w332) -> (error out=w336:errorcluster)  [unwired: 1 in, 1 out]
          n106 = property class="Ctl"(reference=w337, error in=w336, "Visible"=w331, "Disabled"=w327, "Value"=w332) -> (error out=w333:errorcluster)  [unwired: 1 out]
          n107 = property class="Ctl"(reference=w330, error in=w333, "Visible"=w331, "Disabled"=w327, "Value"=w332) -> (error out=w334:errorcluster)  [unwired: 1 out]
          n108 = property class="Ctl"(reference=w329, error in=w334, "Visible"=w331, "Disabled"=w327, "Value"=w332) -> (error out=w326:errorcluster)  [unwired: 1 out]
        }
        frame Default {
          w343 = u8 1 ("Disabled")
          w347 = TRUE
          # "disable normal controls\nif 'default'"
          n109 = To Variant(anything=FALSE) -> (Variant=w348:variant)
          n110 = property class="Ctl"(reference=w354, "Visible"=w347, "Disabled"=w343, "Value"=w348) -> (error out=w352:errorcluster)  [unwired: 1 in, 1 out]
          n111 = property class="Ctl"(reference=w353, error in=w352, "Visible"=w347, "Disabled"=w343, "Value"=w348) -> (error out=w349:errorcluster)  [unwired: 1 out]
          n112 = property class="Ctl"(reference=w346, error in=w349, "Visible"=w347, "Disabled"=w343, "Value"=w348) -> (error out=w350:errorcluster)  [unwired: 1 out]
          n113 = property class="Ctl"(reference=w345, error in=w350, "Visible"=w347, "Disabled"=w343, "Value"=w348) -> (error out=w342:errorcluster)  [unwired: 1 out]
        }
      }
      n114 = call "Check_For_Errors.vi"("Status/Errors in"=w283, "error in"=w282) -> ("Status/Errors out"=w284:refnum<vi>)  [unwired: 9 out]
    }
  }
  "Status/Errors out" <- w18
  "Enabled State Normal" <- w20
  "Enabled State Expert" <- w19
  "DAQ mode value" <- w7
  "Calibration value" <- w2
  n115 = Bundle By Name(cluster=T2 {"Stop program"=FALSE, "Save settings"=FALSE, "Apply settings"=FALSE, "Reset settings"=FALSE, "DAQ mode"=FALSE, "Reset MAS"=FALSE, "Reset SLV"=FALSE, "Local DBase?"=FALSE, "Calibration"=FALSE, "Save settings 2"=FALSE} ("Button values"), "Local DBase?"=w4, "Stop program"=w12, "Save settings"=w11, "Save settings 2"=w1, "Apply settings"=w10, "Reset settings"=w9, "DAQ mode"=w8, "Reset MAS"=w6, "Reset SLV"=w5, "Calibration"=w3) -> (→"Button values":T2)
